vi "Configure File.vi"(7 "Destination File ()":string, 8 "error in (no error)":errorcluster, 9 "Source File ()":string, 10 "File Operation (0: Copy File)":i32(ring) items=["Copy File", "Move File", "Delete File"], 11 "VISA resource name":refnum<visa-resource-name>) -> (0 "error out":errorcluster, 3 "VISA resource name out":refnum<visa-resource-name>)   [LabVIEW 2013, in "Agilent 3446X Series.lvlib"]
doc: "Configures file settings.\n\n<b>Note(s):</b>\nThis vi is not supported for EDU34450A model."
uses:
  <instrlib>/Agilent 3446X Series/Agilent 3446X Series.lvlib
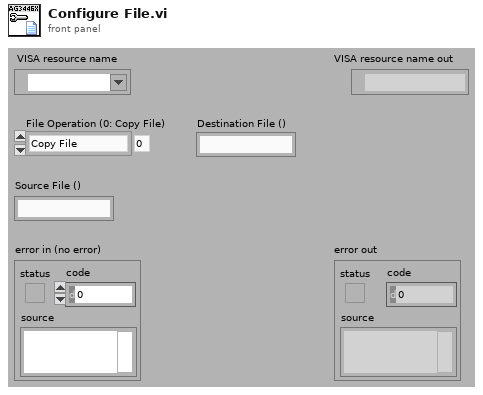
[diagram p1: front panel]
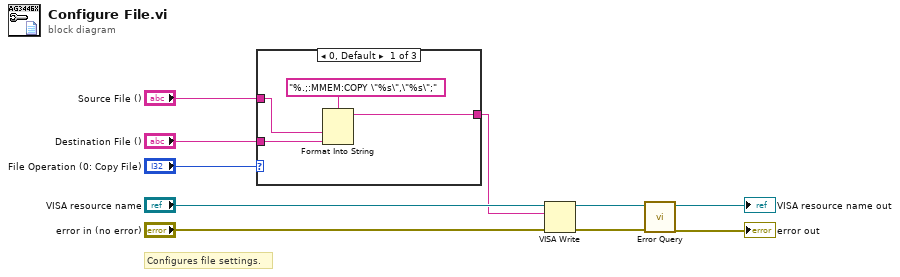
[diagram p0: block diagram]
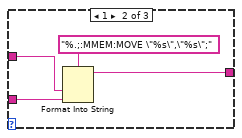
[diagram p2: hidden frame]
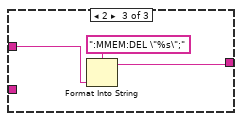
[diagram p3: hidden frame]
diagram:
  # "Configures file settings."
  n1 = case shown="0, Default" "File Operation (0: Copy File)" {
    tunnel: "Source File ()" -> [w14 w17 w20]
    tunnel: "Destination File ()" -> [w11 w15 _]
    tunnel: [w12 w16 w19] -> w1
    frame 0, Default {
      n2 = Format Into String(format string="%.;:MMEM:COPY \"%s\",\"%s\";", w14, w11) -> (resulting string=w12:string)  [unwired: 2 in, 1 out]
    }
    frame 1 {
      n3 = Format Into String(format string="%.;:MMEM:MOVE \"%s\",\"%s\";", w17, w15) -> (resulting string=w16:string)  [unwired: 2 in, 1 out]
    }
    frame 2 {
      n4 = Format Into String(format string=":MMEM:DEL \"%s\";", w20) -> (resulting string=w19:string)  [unwired: 2 in, 1 out]
    }
  }
  n5 = VISA Write(VISA resource name="VISA resource name", write buffer=w1, error in (no error)="error in (no error)") -> (VISA resource name out=w8:refnum<visa-resource-name>, error out=w7:errorcluster)  [unwired: 1 out]
  n6 = call <instrlib>:"Error Query.vi"("error in (no error)"=w7, "VISA resource name"=w8) -> ("error out"=→"error out":errorcluster, "VISA resource name out"=→"VISA resource name out":refnum<visa-resource-name>)  [unwired: 8 out]
